vi "GetLable9550.vi"() -> (0 "字符串":string)   [LabVIEW 2018]
uses:
  <vilib>/Utility/miscctls.llb/LVBoundsTypeDef.ctl
  <vilib>/picture/picture.llb/Draw 1-Bit Pixmap.vi
panel:
  out "长度":i32
  out "二维图片":picture
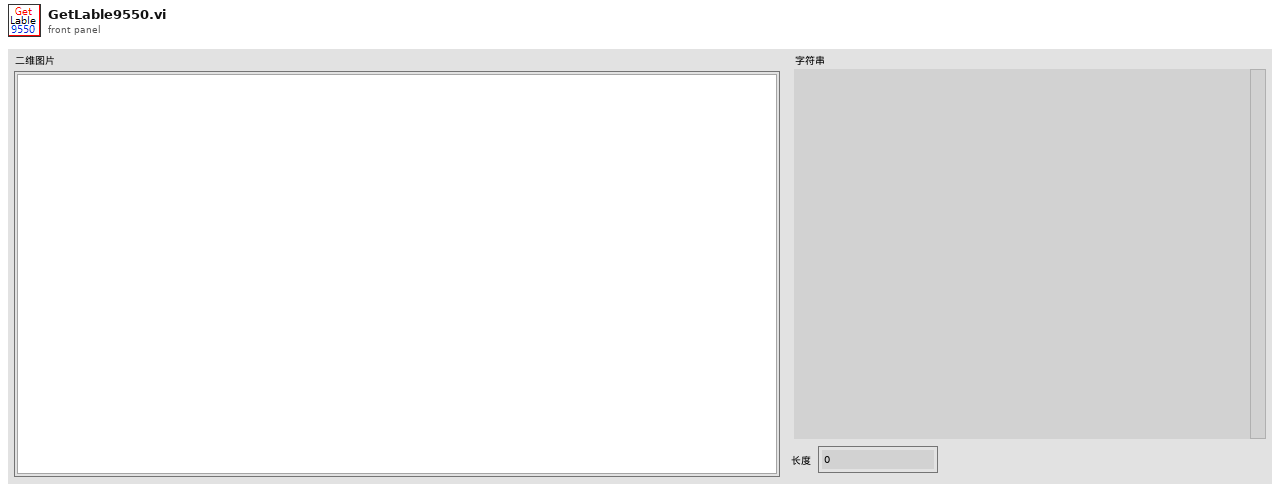
[diagram p1: front panel]
types:
  T1 = cluster{"left":i16, "top":i16, "right":i16, "bottom":i16}
  T2 = typedef "LVBoundsTypeDef.ctl" = cluster{"Width":u32, "Height":u32}
  T3 = enum16{"User-specified Font", "Application Font", "System Font", "Dialog Font"}
  T4 = cluster{"Font Name:":string, "Size":i16, "Strikeout?":bool, "Italic?":bool, "Underline?":bool, "Outline?":bool, "Shadow?":bool, "Bold?":bool}
  T5 = typedef "imagedata.ctl" = cluster{"image type":i32, "image depth":i32, "image":u8[], "mask":u8[], "colors":u32[], "Rectangle":cluster{"left":i16, "top":i16, "right":i16, "bottom":i16}}
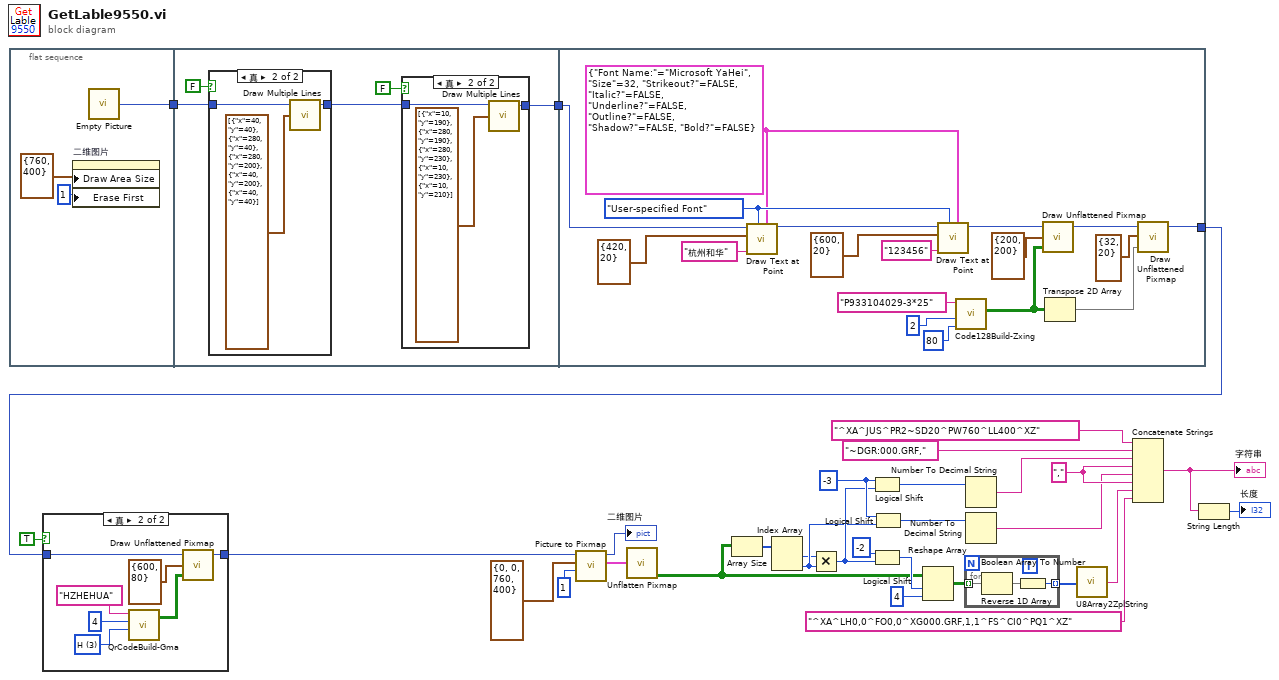
[diagram p0: block diagram]
diagram:
  w14 = ","
  w21 = -3 ("y")
  n1 = flat-sequence {
    tunnel: [w32] -> w30
    tunnel: w30 -> [w36]
    tunnel: [w35] -> w3
    tunnel: w3 -> [w63]
    tunnel: [w53] -> w2
    frame #0 {
      n2 = property on="二维图片" class="Pict"("Draw Area Size"=T2 {"Width"=760, "Height"=400} ("绘图区域大小"), "Erase First"=u8 1 ("画前清除图片")) -> ()  [unwired: 2 in, 2 out]
      n3 = call "Empty Picture"() -> ("empty picture"=w32:picture)
    }
    frame #1 {
      n4 = case shown="真" FALSE {
        tunnel: [w40 w43] -> w39
        tunnel: w36 -> [w40 w41]
        frame False {
        }
        frame True {
          n5 = call <vilib>:"Draw Multiple Lines.vi"("picture"=w41, "line endpoints"=cluster{"x":i16, "y":i16}[] [{"x"=40, "y"=40}, {"x"=280, "y"=40}, {"x"=280, "y"=200}, {"x"=40, "y"=200}, {"x"=40, "y"=40}]) -> ("new picture"=w43:picture)  [unwired: 7 in]
        }
      }
      n6 = case shown="真" FALSE {
        tunnel: w39 -> [w44 w47]
        tunnel: [w44 w46] -> w35
        frame False {
        }
        frame True {
          n7 = call <vilib>:"Draw Multiple Lines.vi"("picture"=w47, "line endpoints"=cluster{"x":i16, "y":i16}[] [{"x"=10, "y"=190}, {"x"=280, "y"=190}, {"x"=280, "y"=230}, {"x"=10, "y"=230}, {"x"=10, "y"=210}]) -> ("new picture"=w46:picture)  [unwired: 7 in]
        }
      }
    }
    frame #2 {
      w60 = T3."User-specified Font" ("desired font(Application)")
      w59 = T4 {"Font Name:"="Microsoft YaHei", "Size"=32, "Strikeout?"=FALSE, "Italic?"=FALSE, "Underline?"=FALSE, "Outline?"=FALSE, "Shadow?"=FALSE, "Bold?"=FALSE} ("[user-specified font]")
      n8 = call <vilib>:"Draw Text at Point.vi"("[user-specified font]"=w59, "desired font(Application)"=w60, "text"="杭州和华", "origin"=cluster{"x":i16, "y":i16} {"x"=420, "y"=20}, "picture"=w63) -> ("new picture"=w61:picture)  [unwired: 5 in, 1 out]
      n9 = call <vilib>:"Draw Text at Point.vi"("[user-specified font]"=w59, "desired font(Application)"=w60, "text"="123456", "origin"=cluster{"x":i16, "y":i16} {"x"=600, "y"=20}, "picture"=w61) -> ("new picture"=w52:picture)  [unwired: 5 in, 1 out]
      n10 = call "Code128Build-Zxing.vi"("ScaleY"=u8 80, "ScaleX"=u8 2, "Text"="P933104029-3*25") -> ("out Array"=w49:bool[][])  [unwired: 2 in]
      n11 = call-poly <vilib>:"Draw Unflattened Pixmap.vi"("picture"=w52, "top left point(0, 0)"=cluster{"x":i16, "y":i16} {"x"=200, "y"=200}, "data"=w49) -> ("new picture"=w51:picture)  [unwired: 6 in]
      n12 = Transpose 2D Array(2D array=w49) -> (transposed array=w50:bool[][])
      n13 = call-poly <vilib>:"Draw Unflattened Pixmap.vi"("picture"=w51, "top left point(0, 0)"=cluster{"x":i16, "y":i16} {"x"=32, "y"=20}, "data"=w50) -> ("new picture"=w53:picture)  [unwired: 6 in]
    }
  }
  n14 = case shown="真" TRUE {
    tunnel: w2 -> [w66 w69]
    tunnel: [w66 w68] -> w29
    frame False {
    }
    frame True {
      w67 = 3 items=["L", "M", "Q", "H"] ("ErrorCorrectLevel")
      n15 = call "QrCodeBuild-Gma.vi"("ErrorCorrectLevel"=w67, "Scale(4)"=u8 4 ("Scale"), "Text"="HZHEHUA") -> ("out Array"=w73:bool[][])  [unwired: 2 in]
      n16 = call-poly <vilib>:"Draw Unflattened Pixmap.vi"("picture"=w69, "top left point(0, 0)"=cluster{"x":i32, "y":i32} {"x"=600, "y"=80} ("position"), "data"=w73) -> ("new picture"=w68:picture)  [unwired: 6 in]
    }
  }
  n17 = call <vilib>:"Picture to Pixmap.vi"("depth"=1, "rect"=T1 {"left"=0, "top"=0, "right"=760, "bottom"=400}, "picture"=w29) -> ("image data"=w28:T5, "new picture"=→"二维图片":picture)  [unwired: 7 in]
  n18 = call <vilib>:"Unflatten Pixmap.vi"("image data"=w28) -> ("1-bit pixmap"=w1:bool[][])  [unwired: 4 in, 6 out]
  n19 = Array Size(array=w1) -> (size(s)=w5:i32[])
  n20 = Index Array(array=w5) -> (element #1=w6:i32, element #2=w17:i32)  [unwired: 2 in]
  n21 = Multiply(x=w6, y=w17) -> (x*y=w20:i32)
  n22 = Logical Shift(y=w21, x=w20) -> (x << y=w19:i32)
  n23 = Logical Shift(y=i16 -2, x=w20) -> (x << y=w16:i32)
  n24 = Logical Shift(y=w21, x=w17) -> (x << y=w18:i32)
  n25 = Reshape Array(w1, w16, 4 ("维数大小")) -> (w7:bool[][])
  n26 = for {
    tunnel: w7 -> [w76] mode=indexing
    tunnel: [w74] -> w22 mode=indexing
    n27 = Reverse 1D Array(array=w76) -> (reversed array=w75:bool[])
    n28 = Boolean Array To Number ("布尔数组至数值转换")(Boolean array=w75) -> (number=w74:u8)
  }
  n29 = Number To Decimal String(number=w19) -> (decimal integer string=w10:string)  [unwired: 1 in]
  n30 = Number To Decimal String(number=w18) -> (decimal integer string=w11:string)  [unwired: 1 in]
  n31 = call "U8Array2ZplString.vi"("in Array"=w22) -> ("字符串"=w23:string)
  n32 = Concatenate Strings("^XA^JUS^PR2~SD20^PW760^LL400^XZ", "~DGR:000.GRF,", w10, w14, w11, w14, w23, "^XA^LH0,0^FO0,0^XG000.GRF,1,1^FS^CI0^PQ1^XZ") -> (w4:string)
  "字符串" <- w4
  n33 = String Length(string=w4) -> (length=→"长度":i32)
